vi "VI Tree.vi"() -> ()   [LabVIEW 2021, in "Pfeiffer Vacuum.lvlib"]
doc: "Pfeiffer Vacuum Tree"
uses:
  <instrlib>/Pfeiffer Vacuum/Pfeiffer Vacuum.lvlib
panel:
  in  "choise":T1(ring)=enum."DigiLine gauges"
  # "SEE DIAGRAM\nFOR VI TREE.\n\nTurbopumps\nOnTool DryPump\nIntegrated Sensors\nDIGILINE Gauges\nActiveLine (TPG36x)\nHandheld Vacuum Gauge\nHLT 5xx\nMiniTest\nASM 340\nDiphragm Pumps\nHiLobe\nModulLine (TPG500)\nHiScroll"
  # "Pfeiffer Vacuum GmbH \n\nBerliner Strasse 43 . D-35614 Asslar\nTel.: +49 (0) 6441 802-0\n Fax: +49 (0) 6441 802-1202\nwww.pfeiffer-vacuum.de"
  # "Version 2021"
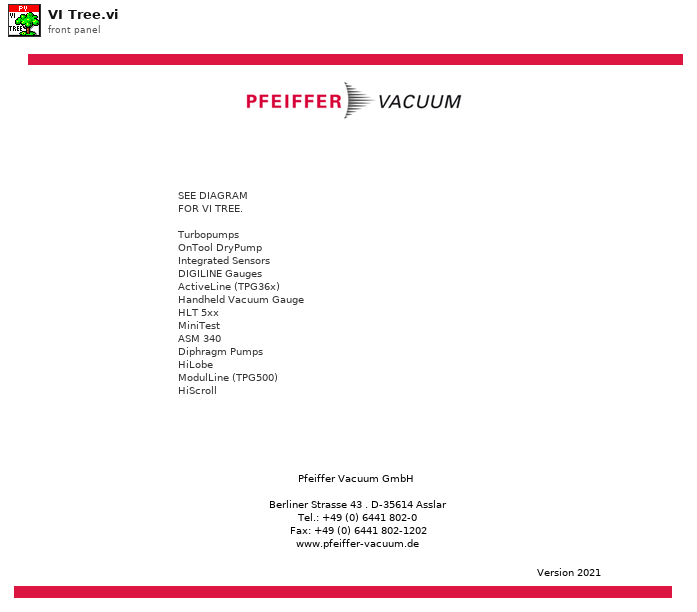
[diagram p1: front panel]
types:
  T1 = enum16{"Turbopump", "Integrated sensors", "OnTool DryPump", "DigiLine gauges", "ModulLine TPG500", "ActiveLine gauges TPG36x", "Handheld vacuum gauge", "HLT 5xx", "MiniTest", "ASM 340", "Diaphragm pumps", "HiLobe", "HiScroll"}
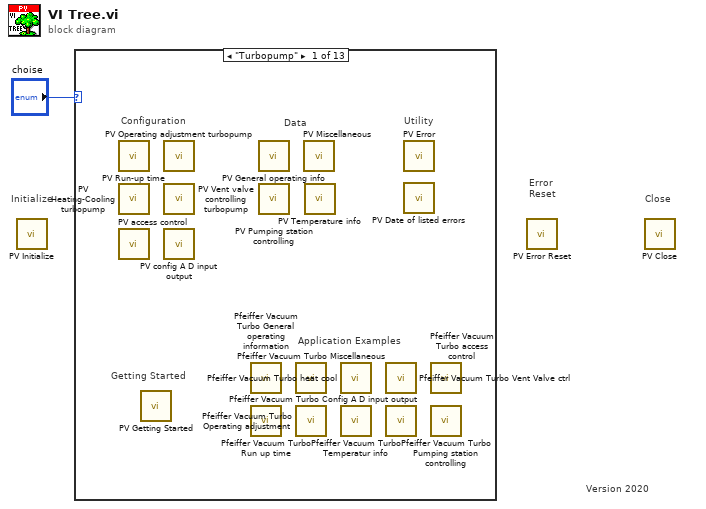
[diagram p0: block diagram]
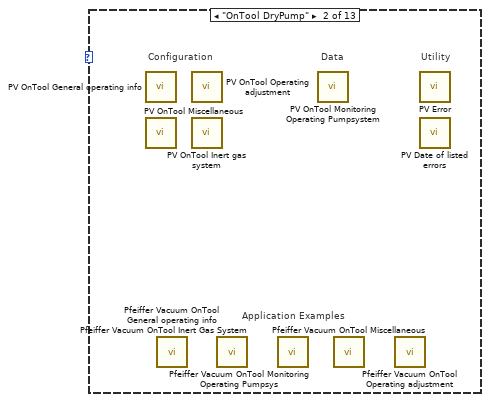
[diagram p2: hidden frame]
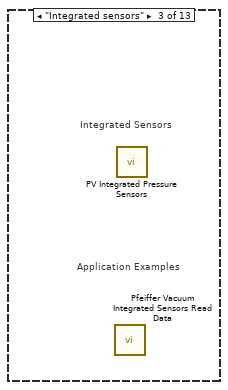
[diagram p3: hidden frame]
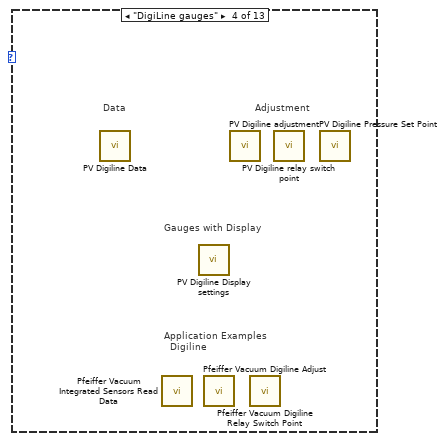
[diagram p4: hidden frame]
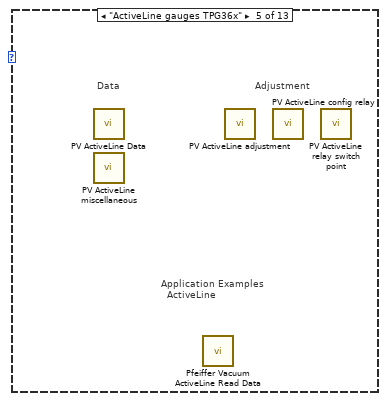
[diagram p5: hidden frame]
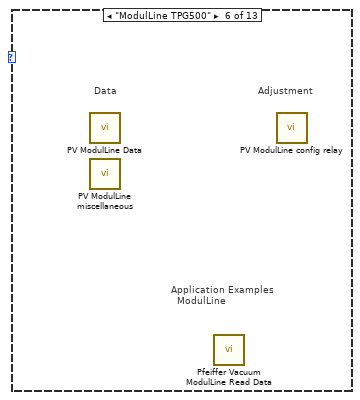
[diagram p6: hidden frame]
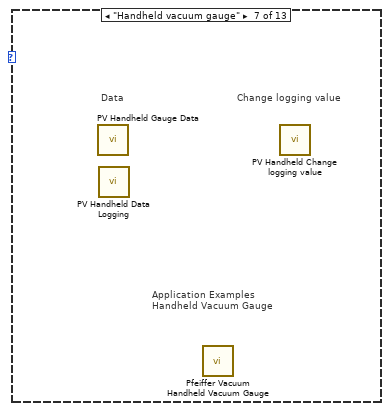
[diagram p7: hidden frame]
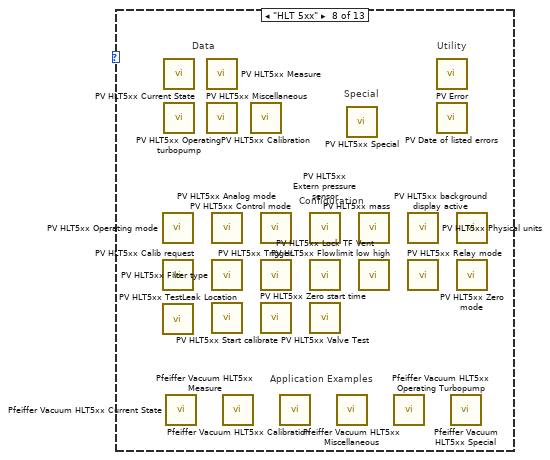
[diagram p8: hidden frame]
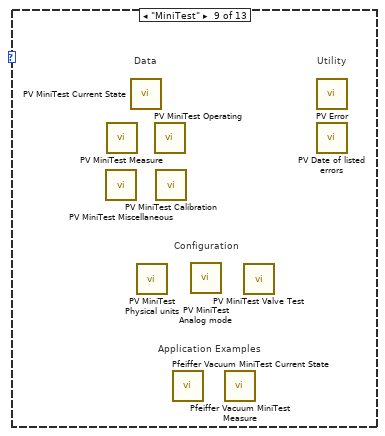
[diagram p9: hidden frame]
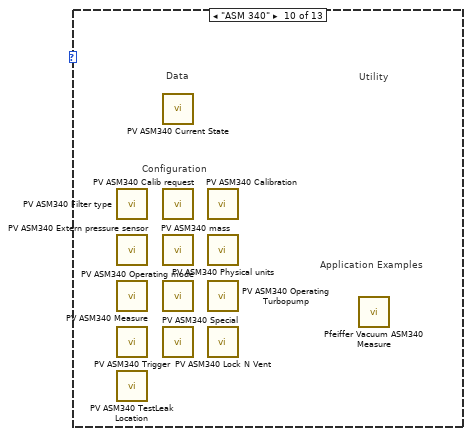
[diagram p10: hidden frame]
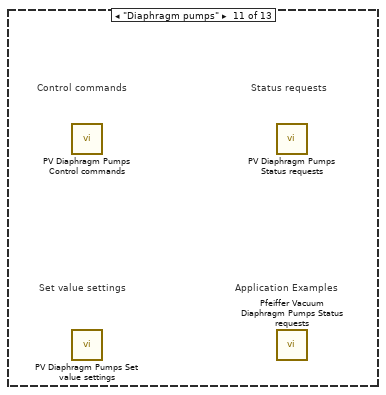
[diagram p11: hidden frame]
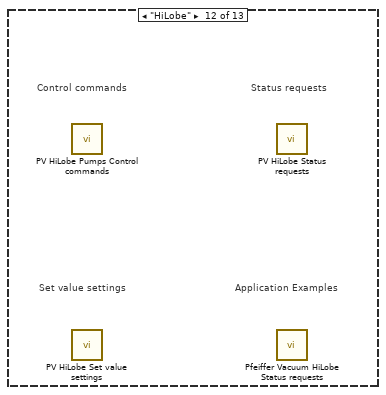
[diagram p12: hidden frame]
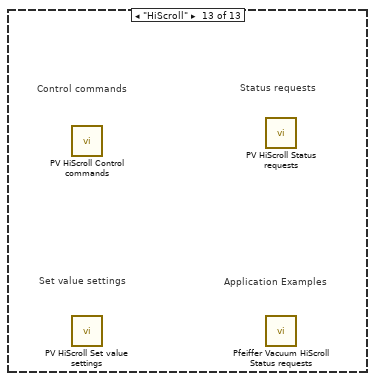
[diagram p13: hidden frame]
diagram:
  # "Error\nReset"
  # "Initialize"
  # "Version 2020"
  # "Close"
  n1 = call <instrlib>:"PV Initialize.vi"() -> ()  [unwired: 10 in, 2 out]
  n2 = case shown="\"Turbopump\"" "choise" {
    frame "Turbopump" {
      # "Getting Started"
      # "Data"
      # "Application Examples"
      # "Utility"
      # "Configuration"
      n3 = call <instrlib>:"PV Run-up time.vi"() -> ()  [unwired: 9 in, 3 out]
      n4 = call <instrlib>:"PV Heating-Cooling turbopump.vi"() -> ()  [unwired: 9 in, 3 out]
      n5 = call <instrlib>:"PV access control.vi"() -> ()  [unwired: 8 in, 3 out]
      n6 = call <instrlib>:"PV Getting Started.vi"() -> ()  [unwired: 13 in, 7 out]
      n7 = call <instrlib>:"PV Operating adjustment turbopump.vi"() -> ()  [unwired: 9 in, 3 out]
      n8 = call <instrlib>:"PV Vent valve controlling turbopump.vi"() -> ()  [unwired: 9 in, 3 out]
      n9 = call <instrlib>:"PV config A D input output.vi"() -> ()  [unwired: 9 in, 3 out]
      n10 = call <instrlib>:"Pfeiffer Vacuum Turbo General operating information.vi"() -> ()  [unwired: 10 in, 2 out]
      n11 = call <instrlib>:"Pfeiffer Vacuum Turbo Run up time.vi"() -> ()  [unwired: 10 in, 2 out]
      n12 = call <instrlib>:"PV General operating info.vi"() -> ()  [unwired: 9 in, 3 out]
      n13 = call <instrlib>:"PV Pumping station controlling.vi"() -> ()  [unwired: 9 in, 3 out]
      n14 = call <instrlib>:"Pfeiffer Vacuum Turbo Miscellaneous.vi"() -> ()  [unwired: 10 in, 2 out]
      n15 = call <instrlib>:"Pfeiffer Vacuum Turbo Operating adjustment.vi"() -> ()  [unwired: 10 in, 2 out]
      n16 = call <instrlib>:"PV Miscellaneous.vi"() -> ()  [unwired: 9 in, 3 out]
      n17 = call <instrlib>:"PV Temperature info.vi"() -> ()  [unwired: 13 in, 3 out]
      n18 = call <instrlib>:"Pfeiffer Vacuum Turbo heat cool.vi"() -> ()  [unwired: 10 in, 2 out]
      n19 = call <instrlib>:"Pfeiffer Vacuum Turbo Temperatur info.vi"() -> ()  [unwired: 10 in, 2 out]
      n20 = call <instrlib>:"Pfeiffer Vacuum Turbo Vent Valve ctrl.vi"() -> ()  [unwired: 10 in, 2 out]
      n21 = call <instrlib>:"Pfeiffer Vacuum Turbo Config A D input output.vi"() -> ()  [unwired: 10 in, 2 out]
      n22 = call <instrlib>:"PV Error.vi"() -> ()  [unwired: 8 in, 4 out]
      n23 = call <instrlib>:"PV Date of listed errors.vi"() -> ()  [unwired: 13 in, 3 out]
      n24 = call <instrlib>:"Pfeiffer Vacuum Turbo access control.vi"() -> ()  [unwired: 10 in, 2 out]
      n25 = call <instrlib>:"Pfeiffer Vacuum Turbo Pumping station controlling.vi"() -> ()  [unwired: 10 in, 2 out]
    }
    frame "OnTool DryPump" {
      # "Utility"
      # "Data"
      # "Configuration"
      # "Application Examples"
      n26 = call <instrlib>:"PV OnTool General operating info.vi"() -> ()  [unwired: 13 in, 3 out]
      n27 = call <instrlib>:"PV OnTool Miscellaneous.vi"() -> ()  [unwired: 9 in, 3 out]
      n28 = call <instrlib>:"Pfeiffer Vacuum OnTool General operating info.vi"() -> ()  [unwired: 10 in, 2 out]
      n29 = call <instrlib>:"PV OnTool Operating adjustment.vi"() -> ()  [unwired: 9 in, 3 out]
      n30 = call <instrlib>:"PV OnTool Inert gas system.vi"() -> ()  [unwired: 9 in, 3 out]
      n31 = call <instrlib>:"Pfeiffer Vacuum OnTool Inert Gas System.vi"() -> ()  [unwired: 10 in, 2 out]
      n32 = call <instrlib>:"Pfeiffer Vacuum OnTool Monitoring Operating Pumpsys.vi"() -> ()  [unwired: 10 in, 2 out]
      n33 = call <instrlib>:"PV OnTool Monitoring Operating Pumpsystem.vi"() -> ()  [unwired: 9 in, 3 out]
      n34 = call <instrlib>:"Pfeiffer Vacuum OnTool Miscellaneous.vi"() -> ()  [unwired: 10 in, 2 out]
      n35 = call <instrlib>:"Pfeiffer Vacuum OnTool Operating adjustment.vi"() -> ()  [unwired: 10 in, 2 out]
      n36 = call <instrlib>:"PV Error.vi"() -> ()  [unwired: 8 in, 4 out]
      n37 = call <instrlib>:"PV Date of listed errors.vi"() -> ()  [unwired: 13 in, 3 out]
    }
    frame "Integrated sensors" {
      # "Application Examples"
      # "Integrated Sensors"
      n38 = call <instrlib>:"Pfeiffer Vacuum Integrated Sensors Read Data.vi"() -> ()  [unwired: 10 in, 2 out]
      n39 = call <instrlib>:"PV Integrated Pressure Sensors.vi"() -> ()  [unwired: 9 in, 3 out]
    }
    frame "DigiLine gauges" {
      # "Gauges with Display"
      # "Adjustment"
      # "Data"
      # "Application Examples\n  Digiline"
      n40 = call <instrlib>:"PV Digiline Data.vi"() -> ()  [unwired: 9 in, 3 out]
      n41 = call <instrlib>:"Pfeiffer Vacuum Integrated Sensors Read Data.vi"() -> ()  [unwired: 10 in, 2 out]
      n42 = call <instrlib>:"PV Digiline Display settings.vi"() -> ()  [unwired: 9 in, 3 out]
      n43 = call <instrlib>:"Pfeiffer Vacuum Digiline Adjust.vi"() -> ()  [unwired: 10 in, 2 out]
      n44 = call <instrlib>:"PV Digiline adjustment.vi"() -> ()  [unwired: 9 in, 3 out]
      n45 = call <instrlib>:"Pfeiffer Vacuum Digiline Relay Switch Point.vi"() -> ()  [unwired: 10 in, 2 out]
      n46 = call <instrlib>:"PV Digiline relay switch point.vi"() -> ()  [unwired: 9 in, 3 out]
      n47 = call <instrlib>:"PV Digiline Pressure Set Point.vi"() -> ()  [unwired: 10 in, 2 out]
    }
    frame "ActiveLine gauges TPG36x" {
      # "Application Examples\n  ActiveLine"
      # "Adjustment"
      # "Data"
      n48 = call <instrlib>:"PV ActiveLine Data.vi"() -> ()  [unwired: 9 in, 3 out]
      n49 = call <instrlib>:"PV ActiveLine miscellaneous.vi"() -> ()  [unwired: 9 in, 3 out]
      n50 = call <instrlib>:"Pfeiffer Vacuum ActiveLine Read Data.vi"() -> ()  [unwired: 10 in, 2 out]
      n51 = call <instrlib>:"PV ActiveLine adjustment.vi"() -> ()  [unwired: 9 in, 3 out]
      n52 = call <instrlib>:"PV ActiveLine config relay.vi"() -> ()  [unwired: 9 in, 3 out]
      n53 = call <instrlib>:"PV ActiveLine relay switch point.vi"() -> ()  [unwired: 9 in, 3 out]
    }
    frame "ModulLine TPG500" {
      # "Adjustment"
      # "Application Examples\n  ModulLine"
      # "Data"
      n54 = call <instrlib>:"PV ModulLine Data.vi"() -> ()  [unwired: 9 in, 3 out]
      n55 = call <instrlib>:"PV ModulLine miscellaneous.vi"() -> ()  [unwired: 9 in, 3 out]
      n56 = call <instrlib>:"Pfeiffer Vacuum ModulLine Read Data.vi"() -> ()  [unwired: 10 in, 2 out]
      n57 = call <instrlib>:"PV ModulLine config relay.vi"() -> ()  [unwired: 9 in, 3 out]
    }
    frame "Handheld vacuum gauge" {
      # "Application Examples\nHandheld Vacuum Gauge"
      # "Data"
      # "Change logging value"
      n58 = call <instrlib>:"PV Handheld Gauge Data.vi"() -> ()  [unwired: 9 in, 3 out]
      n59 = call <instrlib>:"PV Handheld Data Logging.vi"() -> ()  [unwired: 9 in, 3 out]
      n60 = call <instrlib>:"Pfeiffer Vacuum Handheld Vacuum Gauge.vi"() -> ()  [unwired: 10 in, 2 out]
      n61 = call <instrlib>:"PV Handheld Change logging value.vi"() -> ()  [unwired: 8 in, 4 out]
    }
    frame "HLT 5xx" {
      # "Data"
      # "Configuration"
      # "Special"
      # "Application Examples"
      # "Utility"
      n62 = call <instrlib>:"PV HLT5xx Operating mode.vi"() -> ()  [unwired: 8 in, 4 out]
      n63 = call <instrlib>:"PV HLT5xx Calib request.vi"() -> ()  [unwired: 8 in, 4 out]
      n64 = call <instrlib>:"PV HLT5xx TestLeak Location.vi"() -> ()  [unwired: 8 in, 4 out]
      n65 = call <instrlib>:"PV HLT5xx Current State.vi"() -> ()  [unwired: 8 in, 4 out]
      n66 = call <instrlib>:"PV HLT5xx Operating turbopump.vi"() -> ()  [unwired: 9 in, 3 out]
      n67 = call <instrlib>:"Pfeiffer Vacuum HLT5xx Current State.vi"() -> ()  [unwired: 10 in, 2 out]
      n68 = call <instrlib>:"PV HLT5xx Measure.vi"() -> ()  [unwired: 9 in, 3 out]
      n69 = call <instrlib>:"PV HLT5xx Miscellaneous.vi"() -> ()  [unwired: 9 in, 3 out]
      n70 = call <instrlib>:"PV HLT5xx Analog mode.vi"() -> ()  [unwired: 7 in, 5 out]
      n71 = call <instrlib>:"PV HLT5xx Filter type.vi"() -> ()  [unwired: 8 in, 4 out]
      n72 = call <instrlib>:"PV HLT5xx Start calibrate.vi"() -> ()  [unwired: 9 in, 3 out]
      n73 = call <instrlib>:"Pfeiffer Vacuum HLT5xx Measure.vi"() -> ()  [unwired: 10 in, 2 out]
      n74 = call <instrlib>:"PV HLT5xx Calibration.vi"() -> ()  [unwired: 12 in, 4 out]
      n75 = call <instrlib>:"PV HLT5xx Control mode.vi"() -> ()  [unwired: 8 in, 4 out]
      n76 = call <instrlib>:"PV HLT5xx Trigger.vi"() -> ()  [unwired: 9 in, 3 out]
      n77 = call <instrlib>:"PV HLT5xx Zero start time.vi"() -> ()  [unwired: 8 in, 4 out]
      n78 = call <instrlib>:"Pfeiffer Vacuum HLT5xx Calibration.vi"() -> ()  [unwired: 13 in, 3 out]
      n79 = call <instrlib>:"PV HLT5xx Extern pressure sensor.vi"() -> ()  [unwired: 8 in, 4 out]
      n80 = call <instrlib>:"PV HLT5xx Lock TF Vent.vi"() -> ()  [unwired: 8 in, 4 out]
      n81 = call <instrlib>:"PV HLT5xx Valve Test.vi"() -> ()  [unwired: 7 in, 5 out]
      n82 = call <instrlib>:"Pfeiffer Vacuum HLT5xx Miscellaneous.vi"() -> ()  [unwired: 10 in, 2 out]
      n83 = call <instrlib>:"PV HLT5xx Special.vi"() -> ()  [unwired: 9 in, 3 out]
      n84 = call <instrlib>:"PV HLT5xx mass.vi"() -> ()  [unwired: 8 in, 4 out]
      n85 = call <instrlib>:"PV HLT5xx Flowlimit low high.vi"() -> ()  [unwired: 13 in, 3 out]
      n86 = call <instrlib>:"Pfeiffer Vacuum HLT5xx Operating Turbopump.vi"() -> ()  [unwired: 10 in, 2 out]
      n87 = call <instrlib>:"PV HLT5xx Physical units.vi"() -> ()  [unwired: 7 in, 5 out]
      n88 = call <instrlib>:"PV HLT5xx Relay mode.vi"() -> ()  [unwired: 7 in, 5 out]
      n89 = call <instrlib>:"PV Error.vi"() -> ()  [unwired: 8 in, 4 out]
      n90 = call <instrlib>:"PV Date of listed errors.vi"() -> ()  [unwired: 13 in, 3 out]
      n91 = call <instrlib>:"Pfeiffer Vacuum HLT5xx Special.vi"() -> ()  [unwired: 10 in, 2 out]
      n92 = call <instrlib>:"PV HLT5xx background display active.vi"() -> ()  [unwired: 8 in, 4 out]
      n93 = call <instrlib>:"PV HLT5xx Zero mode.vi"() -> ()  [unwired: 8 in, 4 out]
    }
    frame "MiniTest" {
      # "Application Examples"
      # "Configuration"
      # "Data"
      # "Utility"
      n94 = call <instrlib>:"PV MiniTest Miscellaneous.vi"() -> ()  [unwired: 9 in, 3 out]
      n95 = call <instrlib>:"PV MiniTest Measure.vi"() -> ()  [unwired: 9 in, 3 out]
      n96 = call <instrlib>:"PV MiniTest Current State.vi"() -> ()  [unwired: 8 in, 4 out]
      n97 = call <instrlib>:"PV MiniTest Physical units.vi"() -> ()  [unwired: 7 in, 5 out]
      n98 = call <instrlib>:"PV MiniTest Operating.vi"() -> ()  [unwired: 9 in, 3 out]
      n99 = call <instrlib>:"PV MiniTest Calibration.vi"() -> ()  [unwired: 13 in, 3 out]
      n100 = call <instrlib>:"Pfeiffer Vacuum MiniTest Current State.vi"() -> ()  [unwired: 9 in, 3 out]
      n101 = call <instrlib>:"PV MiniTest Analog mode.vi"() -> ()  [unwired: 7 in, 5 out]
      n102 = call <instrlib>:"Pfeiffer Vacuum MiniTest Measure.vi"() -> ()  [unwired: 10 in, 2 out]
      n103 = call <instrlib>:"PV MiniTest Valve Test.vi"() -> ()  [unwired: 9 in, 3 out]
      n104 = call <instrlib>:"PV Error.vi"() -> ()  [unwired: 8 in, 4 out]
      n105 = call <instrlib>:"PV Date of listed errors.vi"() -> ()  [unwired: 13 in, 3 out]
    }
    frame "ASM 340" {
      # "Application Examples"
      # "Configuration"
      # "Utility"
      # "Data"
      n106 = call <instrlib>:"PV ASM340 Filter type.vi"() -> ()  [unwired: 8 in, 4 out]
      n107 = call <instrlib>:"PV ASM340 Extern pressure sensor.vi"() -> ()  [unwired: 8 in, 4 out]
      n108 = call <instrlib>:"PV ASM340 Measure.vi"() -> ()  [unwired: 9 in, 3 out]
      n109 = call <instrlib>:"PV ASM340 Trigger.vi"() -> ()  [unwired: 9 in, 3 out]
      n110 = call <instrlib>:"PV ASM340 TestLeak Location.vi"() -> ()  [unwired: 8 in, 4 out]
      n111 = call <instrlib>:"PV ASM340 Current State.vi"() -> ()  [unwired: 8 in, 4 out]
      n112 = call <instrlib>:"PV ASM340 Calib request.vi"() -> ()  [unwired: 8 in, 4 out]
      n113 = call <instrlib>:"PV ASM340 mass.vi"() -> ()  [unwired: 8 in, 4 out]
      n114 = call <instrlib>:"PV ASM340 Operating mode.vi"() -> ()  [unwired: 8 in, 4 out]
      n115 = call <instrlib>:"PV ASM340 Special.vi"() -> ()  [unwired: 9 in, 3 out]
      n116 = call <instrlib>:"PV ASM340 Calibration.vi"() -> ()  [unwired: 12 in, 4 out]
      n117 = call <instrlib>:"PV ASM340 Physical units.vi"() -> ()  [unwired: 7 in, 5 out]
      n118 = call <instrlib>:"PV ASM340 Operating Turbopump.vi"() -> ()  [unwired: 9 in, 3 out]
      n119 = call <instrlib>:"PV ASM340 Lock N Vent.vi"() -> ()  [unwired: 8 in, 4 out]
      n120 = call <instrlib>:"Pfeiffer Vacuum ASM340 Measure.vi"() -> ()  [unwired: 10 in, 2 out]
    }
    frame "Diaphragm pumps" {
      # "Application Examples"
      # "Set value settings"
      # "Control commands"
      # "Status requests"
      n121 = call <instrlib>:"PV Diaphragm Pumps Control commands .vi"() -> ()  [unwired: 9 in, 3 out]
      n122 = call <instrlib>:"PV Diaphragm Pumps Set value settings.vi"() -> ()  [unwired: 9 in, 3 out]
      n123 = call <instrlib>:"PV Diaphragm Pumps Status requests.vi"() -> ()  [unwired: 9 in, 3 out]
      n124 = call <instrlib>:"Pfeiffer Vacuum Diaphragm Pumps Status requests .vi"() -> ()  [unwired: 10 in, 2 out]
    }
    frame "HiLobe" {
      # "Application Examples"
      # "Set value settings"
      # "Control commands"
      # "Status requests"
      n125 = call <instrlib>:"PV HiLobe Pumps Control commands .vi"() -> ()  [unwired: 9 in, 3 out]
      n126 = call <instrlib>:"PV HiLobe Set value settings.vi"() -> ()  [unwired: 9 in, 3 out]
      n127 = call <instrlib>:"PV HiLobe Status requests.vi"() -> ()  [unwired: 9 in, 3 out]
      n128 = call <instrlib>:"Pfeiffer Vacuum HiLobe Status requests.vi"() -> ()  [unwired: 10 in, 2 out]
    }
    frame "HiScroll" {
      # "Application Examples"
      # "Status requests"
      # "Set value settings"
      # "Control commands"
      n129 = call <instrlib>:"PV HiScroll Control commands .vi"() -> ()  [unwired: 9 in, 3 out]
      n130 = call <instrlib>:"PV HiScroll Set value settings.vi"() -> ()  [unwired: 9 in, 3 out]
      n131 = call <instrlib>:"PV HiScroll Status requests.vi"() -> ()  [unwired: 9 in, 3 out]
      n132 = call <instrlib>:"Pfeiffer Vacuum HiScroll Status requests .vi"() -> ()  [unwired: 10 in, 2 out]
    }
  }
  n133 = call <instrlib>:"PV Error Reset.vi"() -> ()  [unwired: 10 in, 2 out]
  n134 = call <instrlib>:"PV Close.vi"() -> ()  [unwired: 15 in, 1 out]
